vi "ni579x Close.vi"(0 "Register Bus":refnum<class "ni579x Register Bus v1 Host.lvclass">, 11 "error in":errorcluster) -> (4 "fpga ref":refnum<k20>, 15 "error out":errorcluster)   [LabVIEW 2015]
doc: "Closes the session to the NI-579x Configuration Design Library by destroying the session to the Register Bus Host library."
uses:
  <instrlib>/ni579x/Register Bus/v1/Host/ni579x Register Bus v1 Host.lvclass
  <vilib>/ErrorRing/Error Ring.xnode
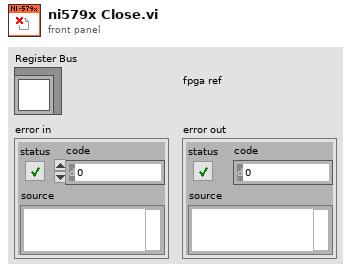
[diagram p1: front panel]
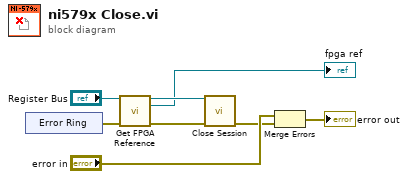
[diagram p0: block diagram]
diagram:
  n1 = xnode "Error Ring"() -> ("error out"=w1:errorcluster)
  n2 = call <instrlib>:"Get FPGA Reference.vi"("session in"="Register Bus", "error in"=w1) -> ("session out"=w6:refnum<class "ni579x Register Bus v1 Host.lvclass">, "fpga ref"=→"fpga ref":refnum<k20>, "error out"=w8:errorcluster)  [unwired: 11 in]
  n3 = call <instrlib>:"Close Session.vi"("session in"=w6, "error in"=w8) -> ("error out"=w4:errorcluster)  [unwired: 13 in]
  n4 = Merge Errors("error in", w4) -> (→"error out":errorcluster)
